vi "FRCts20_Backend_Competition_GET.vi"(6 "Message Attributes":T4, 8 "error in (no error)":errorcluster, 10 "Data":string, 11 "Engine_Refnums":T1) -> (0 "error out":errorcluster)   [LabVIEW 2013]
doc: "Gets all divisions under a selected competition. Called by the competition/division api, and expects a competition name."
uses:
  FRCts20_Backend_Engine.lvlib
  FRCts20_Backend_API/FRCts20_Backend_API_Competition.ctl
  FRCts20_Backend_API/FRCts20_Backend_API.lvlib
  FRCts20_Backend_FGVOperation.ctl
  Dependencies/Keyed Array/KeyedArray.ctl
  Dependencies/Keyed Array/Tools_KeyedArray.lvlib
  Dependencies/AMC/_SubVIs/TypeDefs/Message.ctl
  Dependencies/AMC/AMC.lvlib
  Dependencies/AMC/_SubVIs/TypeDefs/Message Queue.ctl
  <vilib>/addons/database/Connection.llb/Conn ObjectReference.ctl
  <vilib>/addons/database/NI_Database_API.lvlib
  FRCts20_Backend_EngineRefnums.ctl
  INI_Accessor/FRCts20_Backend_INI Controller.lvclass
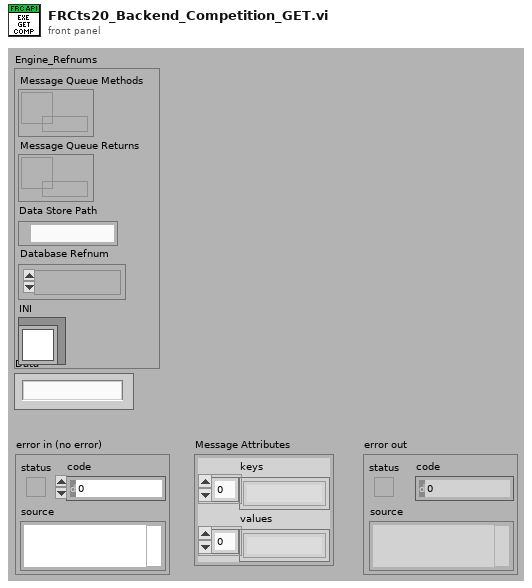
[diagram p1: front panel]
types:
  T1 = typedef "FRCts20_Backend_Engine.lvlib/FRCts20_Backend_EngineRefnums.ctl" = cluster{"Message Queue Methods":T2, "Message Queue Returns":T2, "Data Store Path":path, "Database Refnum":T3, "INI":refnum<class "FRCts20_Backend_INI Controller.lvclass">}
  T2 = typedef "AMC.lvlib/Message Queue.ctl" = refnum<queue>
  T3 = typedef "NI_Database_API.lvlib/Conn ObjectReference.ctl" = refnum<k1>
  T4 = typedef "Tools_KeyedArray.lvlib/KeyedArray.ctl" = cluster{"keys":string[], "values":string[]}
  T5 = typedef "FRCts20_Backend_Engine.lvlib/FRCts20_Backend_FGVOperation.ctl" = enum16{"Initialize", "EnqueueMessage", "EnqueueDataReturn", "FlushMessage", "FlushDataReturn"}
  T6 = typedef "FRCts20_Backend_API.lvlib/FRCts20_Backend_API_Competition.ctl" = cluster{"Name":string, "Start Date":timestamp, "Duration":u8, "Divisions":string[], "APIReturn":string}
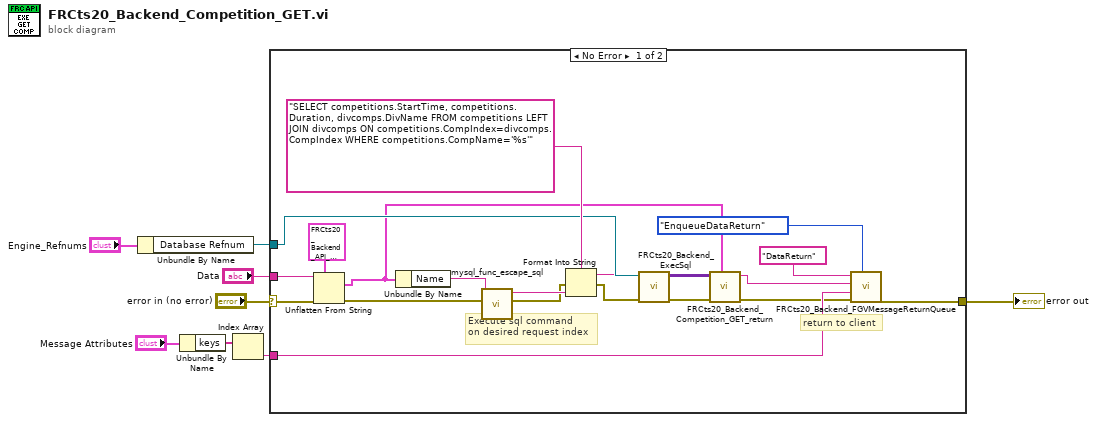
[diagram p0: block diagram]
diagram:
  n1 = Unbundle By Name("Engine_Refnums") -> ("Database Refnum"=w1:T3)
  n2 = Unbundle By Name("Message Attributes") -> ("keys"=w4:string[])
  n3 = Index Array(array=w4) -> (element=w3:string)  [unwired: 1 in]
  n4 = case shown="No Error" "error in (no error)" {
    selector: "error in (no error)" -> [w25 w29]
    tunnel: [w28 w29] -> w7
    tunnel: w1 -> [w15 _]
    tunnel: "Data" -> [w26 _]
    tunnel: w3 -> [w27 _]
    frame No Error {
      # "return to client"
      # "Execute sql command\non desired request index"
      n5 = Unflatten From String(type=T6 {"Name"="", "Start Date"=timestamp(0 s since 1904-01-01), "Duration"=0, "Divisions"=[], "APIReturn"=""} ("Competition"), binary string=w26, error in (no error)=w25) -> (value=w11:T6, error out=w18:errorcluster)  [unwired: 2 in, 1 out]
      n6 = Unbundle By Name(w11) -> ("Name"=w19:string)
      n7 = call "mysql_func_escape_sql.vi"("error in (no error)"=w18, "sqlin"=w19) -> ("error out"=w16:errorcluster, "escaped"=w17:string)  [unwired: 8 in]
      n8 = Format Into String(format string="SELECT competitions.StartTime, competitions.Duration, divcomps.DivName FROM competitions LEFT JOIN divcomps ON competitions.CompIndex=divcomps.CompIndex WHERE competitions.CompName='%s'", error in=w16, w17) -> (resulting string=w13:string, error out=w14:errorcluster)  [unwired: 1 in]
      n9 = call "FRCts20_Backend_ExecSql.vi"("error in (no error)"=w14, "format string"=w13, "Refnum in"=w15) -> ("error out"=w12:errorcluster, "recordset data"=w10:variant[][])  [unwired: 6 in, 1 out]
      n10 = call "FRCts20_Backend_Competition_GET_return.vi"("Competition"=w11, "error in (no error)"=w12, "recordset data"=w10) -> ("error out"=w21:errorcluster, "data string"=w22:string)  [unwired: 7 in]
      n11 = call "FRCts20_Backend_FGVMessageReturnQueue.vi"("Operation"=FRCts20_Backend_FGVOperation."EnqueueDataReturn", "error in (no error)"=w21, "Key"=w27, "Message Value"=w22, "Message Name"="DataReturn") -> ("error out"=w28:errorcluster)  [unwired: 5 in, 1 out]
    }
    frame Error {
    }
  }
  "error out" <- w7
